vi "Message.vi"(3 "error in (no error)":errorcluster, 5 "Message":string) -> (0 "error out":errorcluster)   [LabVIEW 2017]
doc: "Update message on display."
panel:
  in  "Ok":bool
  out "Message":string
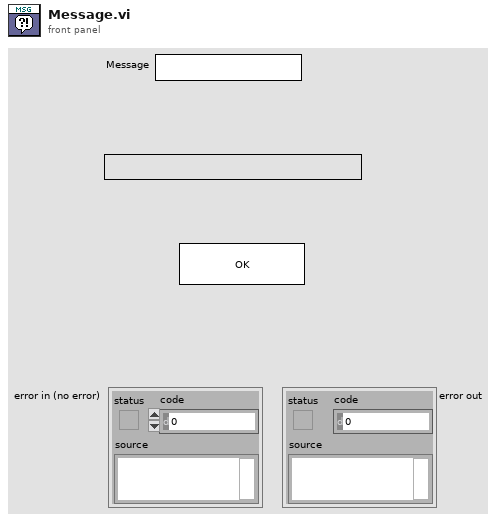
[diagram p1: front panel]
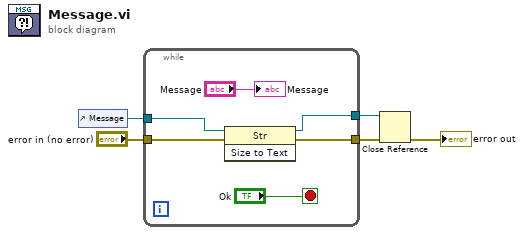
[diagram p0: block diagram]
diagram:
  n1 = control-ref of="Message"() -> (w4:refnum<vi>)
  n2 = while {
    tunnel: "error in (no error)" -> [w8]
    tunnel: [w7] -> w3
    tunnel: w4 -> [w9]
    tunnel: [w6] -> w2
    stop <- "Ok" stop-if-true
    n3 = invoke class="Str" method="Size to Text"(reference=w9, error in=w8) -> (reference out=w6:refnum<vi>, error out=w7:errorcluster)  [unwired: 1 in, 1 out]
    "Message" <- "Message"
  }
  n4 = Close Reference(reference=w2, error in (no error)=w3) -> (error out=→"error out":errorcluster)
